vi "Write Type Name Handling.vi"(8 "error in (no error)":errorcluster, 10 "Type Name Handling":T1, 11 "Flatten To JSON Object in":refnum<class "Generic Object Serializer.lvclass">) -> (0 "error out":errorcluster, 3 "Flatten To JSON Object out":refnum<class "Generic Object Serializer.lvclass">)   [LabVIEW 2017, in "Generic Object Serializer.lvclass"]
uses:
  Generic Object Serializer/Generic Object Serializer.lvclass
  Type Name Handling.ctl
  Generic Object Serializer/Generic Object Serializer.lvclass/Generic Object Serializer.ctl
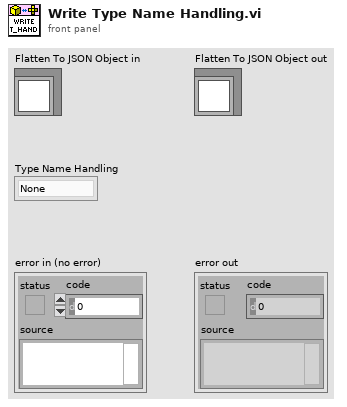
[diagram p1: front panel]
types:
  T1 = typedef "Generic Object Serializer.lvclass/Type Name Handling.ctl" = enum16{"None", "Inline"}
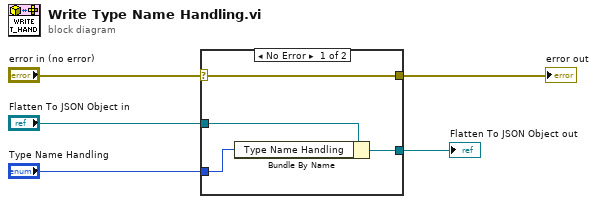
[diagram p0: block diagram]
diagram:
  n1 = case shown="No Error" "error in (no error)" {
    selector: "error in (no error)" -> [w9 w10]
    tunnel: [w9 w10] -> w4
    tunnel: [w7 w11] -> w2
    tunnel: "Flatten To JSON Object in" -> [w8 w11]
    tunnel: "Type Name Handling" -> [w6 _]
    frame No Error {
      n2 = Bundle By Name(cluster=w8, "Type Name Handling"=w6) -> (w7:refnum<class "Generic Object Serializer.lvclass">)
    }
    frame Error {
    }
  }
  "error out" <- w4
  "Flatten To JSON Object out" <- w2
